vi "Check-filter-conditions.vi"(7 "Monitor":bool, 8 "error in":errorcluster, 9 "Value":dbl, 10 "Duration in":u16, 11 "Conditions":T1) -> (0 "error":errorcluster, 1 "Alert?":bool, 2 "Duration":u16)   [LabVIEW 2013, in "CameraVision.lvlib" / "CV-Filter.lvclass"]
doc: "Alert if the value is:\na) not within the min/max limits AND \nb) higher than the minimum threshold AND\nc) this is valid for at least 'duration' samples."
uses:
  CV-Filter.lvclass
  Filter-settings.ctl
  Filter-characteristic.ctl
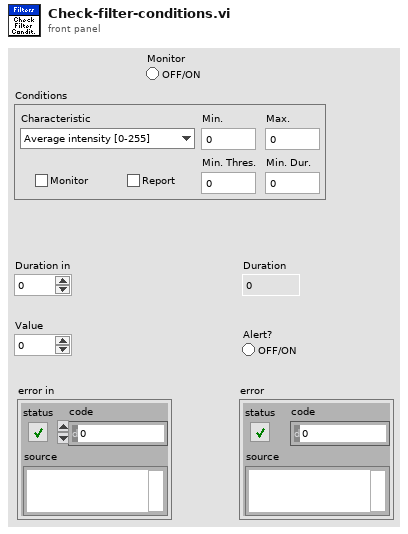
[diagram p1: front panel]
types:
  T1 = typedef "CameraVision.lvlib/CV-Filter.lvclass/Filter-settings.ctl" = cluster{"Characteristic":T2, "Monitor":bool, "Min.":dbl, "Max.":dbl, "Min. Thres.":dbl, "Min. Dur.":u16, "Report":bool}
  T2 = typedef "CameraVision.lvlib/CV-Filter.lvclass/Filter-characteristic.ctl" = enum16{"Average intensity [0-255]", "Peak intensity [0-255]", "Melt-pool size [mm²]", "Melt-pool aspect ratio []", "Melt-pool fragments []", "Melt-pool position X [pixel]", "Melt-pool position Y [pixel]", "Average temperature [°C]", "Max. temperature [°C]", "Min. temperature [°C]", "Std. dev. temperature [°C]"}
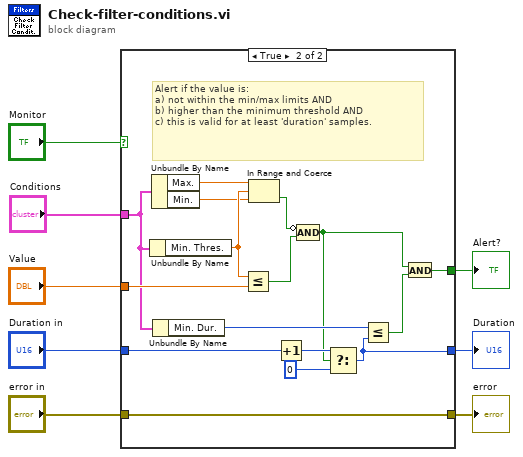
[diagram p0: block diagram]
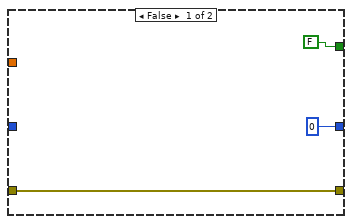
[diagram p2: hidden frame]
diagram:
  n1 = case shown="True" "Monitor" {
    tunnel: "Value" -> [_ w26]
    tunnel: "Duration in" -> [_ w18]
    tunnel: "Conditions" -> [_ w20]
    tunnel: "error in" -> [w9 w27]
    tunnel: [w9 w27] -> w7
    tunnel: [u16 0 ("Duration in") w15] -> w6
    tunnel: [FALSE w12] -> w8
    frame False {
    }
    frame True {
      # "Alert if the value is:\na) not within the min/max limits AND \nb) higher than the minimum threshold AND\nc) this is valid for at least 'duration' samples."
      n2 = Unbundle By Name(w20) -> ("Min. Thres."=w25:dbl)
      n3 = Unbundle By Name(w20) -> ("Max."=w24:dbl, "Min."=w23:dbl)
      n4 = Unbundle By Name(w20) -> ("Min. Dur."=w19:u16)
      n5 = Less Or Equal?(x=w25, y=w26) -> (x <= y?=w21:bool)
      n6 = In Range and Coerce(upper limit=w24, x=w25, lower limit=w23) -> (In Range?=w22:bool)  [unwired: 1 out]
      n7 = Increment(x=w18) -> (x+1=w16:u16)
      n8 = Compound Arithmetic op=AND(invert w22, w21) -> (w13:bool)
      n9 = Select(t=w16, s=w13, f=u16 0) -> (s? t:f=w15:u16)
      n10 = Less Or Equal?(x=w19, y=w15) -> (x <= y?=w14:bool)
      n11 = And(x=w13, y=w14) -> (x .and. y?=w12:bool)
    }
  }
  "Alert?" <- w8
  "error" <- w7
  "Duration" <- w6
